vi "Bertta_v09_5.vi"() -> ()   [LabVIEW 2015]
uses:
  x64/Debug/BERTTA.dll
panel:
  out "TIME array":dbl[](array[numeric])
  out "TEMP array":dbl[](array[numeric])
  out "element":bool
  out "Started:":string
  in  "SHUTDOWN":bool
  in  "MASTER CONTROL":bool
  in  "Tab Control":T1(tab)
  in  "Read Seq":bool
  in  "Save Seq":bool
  in  "Configuration file":path=path "C:/Users/shresplab/Desktop/BerttaConfiguration.lvm" caption="Filename"
  in  "OK Button 2":bool
  out "Boolean":bool
  in  "User (initials)":string
  in  "Project name":string
  in  "Description":string
  out "Output file":string
  out "PUMP 3":bool
  out "Target amount":dbl
  out "Scale weight":dbl
  out "Amount now":dbl
  out "Flow rate":dbl
  out "Time to target":dbl format="%<%H:%M:%S>t"
  out "Current step":dbl
  out "Target amount":dbl
  out "Amount now":dbl
  out "Amount now":dbl
  out "Target amount":dbl
  out "Current step":dbl
  out "Time to target":dbl format="%<%H:%M:%S>t"
  out "Flow rate":dbl
  out "Amount now":dbl
  out "Scale weight":dbl
  out "Target amount":dbl
  out "PUMP 2":bool
  out "Sensor OK 6":bool
  out "Sensor OK 5":bool
  out "Sensor OK 4":bool
  out "Sensor OK 3":bool
  in  "OK Button":bool
  in  "Add comment":string
  out "PUMP 1":bool
  out "Target amount":dbl
  out "Scale weight":dbl
  out "Amount now":dbl
  out "Flow rate":dbl
  out "Time to target":dbl format="%<%H:%M:%S>t"
  out "Current step":dbl
  out "Target amount":dbl
  out "Amount now":dbl
  out "Tr":dbl
  out "Tj in":dbl
  out "Tj out":dbl
  out "T set":dbl
  out "Current step":i32
  out "RPM":dbl
  out "Torque 2":dbl
  out "Waveform Chart 5":dynamicdata(graph)
  out "Waveform Chart 6":dynamicdata(graph)
  out "Waveform Chart 7":dynamicdata(graph)
  in  "Tab Control 2":T2(tab)
  out "Waveform Chart 3":dynamicdata(graph)
  out "Waveform Chart 8":dynamicdata(graph)
  out "Waveform Chart 11":dynamicdata(graph)
  out "Waveform Chart 13":dynamicdata(graph)
  out "Waveform Chart 9":dynamicdata(graph)
  out "Table":string[][](table)=[["14.8.2017 18.06.59", "0,000000", "417,670000", "-0,150000", "1,000000", "22,220000", "23,366837", "23,574959", "23,985852", "23,690000", "240,000000", "4,000000", "0,000000", "397,000000", "-397,000000", "1,000000"], ["14.8.2017 18.07.06", "0,000000", "417,640000", "-0,120000", "1,000000", "22,220000", "23,763115", "23,906257", "23,985694", "23,680000", "240,000000", "4,000000", "0,000000", "397,000000", "-397,000000", "1,000000"], ["14.8.2017 18.07.13", "0,000000", "417,640000", "-0,120000", "1,000000", "22,220000", "23,965922", "24,013440", "23,984906", "23,670000", "240,000000", "4,100000", "3,000000", "397,000000", "-397,000000", "1,000000"], ["14.8.2017 18.07.21", "0,000000", "417,640000", "-0,120000", "1,000000", "22,220000", "23,943860", "23,900110", "23,987113", "23,670000", "240,000000", "4,000000", "0,000000", "397,000000", "-397,000000", "1,000000"], ["14.8.2017 18.07.28", "0,000000", "417,640000", "-0,120000", "1,000000", "22,220000", "23,736328", "23,600018", "23,989004", "23,660000", "240,000000", "4,000000", "0,000000", "397,000000", "-397,000000", "1,000000"], ["14.8.2017 18.07.36", "0,000000", "417,640000", "-0,120000", "1,000000", "22,220000", "23,480910", "23,324538", "23,991053", "23,660000", "240,000000", "4,000000", "0,000000", "397,000000", "-397,000000", "1,000000"], ["14.8.2017 18.07.43", "0,000000", "417,640000", "-0,120000", "2,000000", "22,220000", "23,195579", "23,008270", "23,999093", "23,650000", "240,000000", "4,000000", "0,000000", "397,000000", "-397,000000", "1,000000"], ["14.8.2017 18.07.51", "0,000000", "417,650000", "-417,650000", "1,000000", "22,220000", "22,862541", "22,649021", "24,003979", "23,650000", "240,000000", "4,000000", "0,000000", "397,000000", "-397,000000", "2,000000"], ["14.8.2017 18.07.58", "0,000000", "417,640000", "0,010000", "1,000000", "22,220000", "22,541353", "22,354878", "24,005398", "23,650000", "240,000000", "4,000000", "0,000000", "397,000000", "-397,000000", "1,000000"], ["14.8.2017 18.08.06", "0,000000", "417,640000", "0,010000", "1,000000", "22,220000", "22,347931", "22,253738", "24,007605", "23,640000", "240,000000", "4,100000", "0,000000", "397,000000", "-397,000000", "1,000000"], ["14.8.2017 18.08.13", "0,000000", "417,640000", "0,010000", "1,000000", "22,220000", "22,329030", "22,302102", "24,006028", "23,640000", "240,000000", "4,000000", "0,000000", "395,820000", "-395,820000", "1,000000"], ["14.8.2017 18.08.20", "0,000000", "417,640000", "0,010000", "1,000000", "22,220000", "22,466849", "22,511320", "24,002403", "23,630000", "240,000000", "4,000000", "0,000000", "395,830000", "-0,010000", "1,000000"], ["14.8.2017 18.08.28", "0,000000", "417,640000", "0,010000", "1,000000", "22,220000", "22,707062", "22,835101", "24,000984", "23,620000", "240,000000", "4,000000", "0,000000", "395,830000", "-0,010000", "1,000000"], ["14.8.2017 18.08.35", "0,000000", "417,640000", "0,010000", "1,000000", "22,220000", "23,054104", "23,232979", "24,001299", "23,600000", "240,000000", "4,000000", "0,000000", "395,830000", "-0,010000", "1,000000"], ["14.8.2017 18.08.43", "0,000000", "417,640000", "0,010000", "1,000000", "22,220000", "23,412371", "23,522793", "24,002560", "23,590000", "240,000000", "4,000000", "0,000000", "395,820000", "0,000000", "1,000000"], ["14.8.2017 18.08.51", "0,000000", "417,640000", "0,010000", "1,000000", "22,220000", "23,596247", "23,656125", "24,003821", "23,580000", "240,000000", "4,000000", "0,000000", "395,820000", "0,000000", "1,000000"]]
  in  "Reset":bool
  in  "Numeric 4":dbl=20.0
  in  "Numeric 3":dbl=30.0
  in  "Numeric 2":dbl=40.0
  in  "Numeric 1":dbl=30.0
  in  "Numeric":dbl=20.0
  out "Boolean 12":bool
  out "Boolean 7":bool
  out "Boolean 6":bool
  out "Boolean 5":bool
  out "Boolean 4":bool
  out "Boolean 19":bool
  in  "Numeric 5":dbl=5.0
  in  "Numeric 6":dbl=5.0
  in  "Numeric 7":dbl=5.0
  in  "Numeric 8":dbl=5.0
  in  "T ext / T ext 2":enum32{"External 1", "External 2"}(radio)
  out "Sensor OK":bool
  in  "T fail":dbl=20.0
  in  "?":bool
  in  "T manual setpoint":dbl=20.0
  in  "Lauda port":dbl=9.0
  in  "Manual select":enum32{"Tr", "Tj"}(radio)
  in  "PAUSE":bool
  out "Waveform Chart":dynamicdata(graph)
  out "T external 2":dbl
  out "result":bool
  in  "Port":i32=10
  in  "Radio Buttons 3":enum32{"Reglo Digital", "Reglo Analog", "PAM"}(radio)=enum."Reglo Analog"
  out "Speed":dbl
  out "mA":dbl format="%#_2g"
  in  "Port":i32=15
  out "RPM":dbl format="%#_2g"
  out "Led10 3":bool
  out "Led9 3":bool
  out "Led8 3":bool
  out "Led7 3":bool
  out "Led6 3":bool
  out "Led5 3":bool
  out "Led4 3":bool
  out "Led3 3":bool
  out "Led2 3":bool
  out "Led1 3":bool
  in  "PumpSeq 3":dbl[][](array[numeric])=[[0.0, 0.0, 7.0], [0.0, 0.0, 2.0], [0.0, 0.0, 100.0], [0.0, 0.0, 0.0], [0.0, 0.0, 0.0], [0.0, 0.0, 0.0], [0.0, 0.0, 0.0], [0.0, 0.0, 0.0], [0.0, 0.0, 0.0], [0.0, 0.0, 0.0], [0.0, 1.0, 0.0]]
  in  "?":bool
  out "Flow rate (g/min)":dbl
  out "Scale reading":dbl
  out "Step amount now":dbl
  out "Time to target":dbl format="%<%H:%M:%S>t"
  in  "Grams / min":dbl
  out "Waveform Chart 12":dynamicdata(graph)
  in  "?":bool
  out "Total amount now":dbl
  out "Total time 3":dbl
  out "Total amount target 3":dbl
  out "Led11 3":bool
  in  "Reset 4":bool
  in  "Port":i32=11
  in  "Radio Buttons 2":enum32{"Reglo Digital", "Reglo Analog", "PAM"}(radio)
  out "Speed":dbl
  out "mA":dbl format="%#_2g"
  in  "Port":i32=15
  out "RPM":dbl format="%_4f"
  out "Led10 2":bool
  out "Led9 2":bool
  out "Led8 2":bool
  out "Led7 2":bool
  out "Led6 2":bool
  out "Led5 2":bool
  out "Led4 2":bool
  out "Led3 2":bool
  out "Led2 2":bool
  out "Led1 2":bool
  in  "PumpSeq 2":dbl[][](array[numeric])=[[1.0, 2.0, 7.0], [2.0, 2.0, 2.0], [3.0, 2.0, 100.0], [0.0, 0.0, 0.0], [0.0, 0.0, 0.0], [0.0, 0.0, 0.0], [0.0, 0.0, 0.0], [0.0, 0.0, 0.0], [0.0, 0.0, 0.0], [0.0, 0.0, 0.0], [0.0, 1.0, 0.0]]
  in  "?":bool
  out "Flow rate (g/min)":dbl
  out "Scale reading":dbl
  out "Step amount now":dbl
  out "Time to target":dbl format="%<%H:%M:%S>t"
  in  "Grams / min":dbl
  out "Waveform Chart 10":dynamicdata(graph)
  in  "?":bool
  out "Total amount now":dbl
  out "Total time 2":dbl
  out "Total amount target 2":dbl
  out "Led11 2":bool
  in  "Reset 3":bool
  out "elapsed / step":i32
  out "step_fr":dbl
  in  "Port":i32=12
  in  "Radio Buttons":enum32{"Reglo Digital", "Reglo Analog", "PAM"}(radio)
  out "Speed":dbl
  out "mA":dbl format="%#_2g"
  in  "Port":i32=14
  out "RPM":dbl format="%#_2g"
  out "Led10":bool
  out "Led9":bool
  out "Led8":bool
  out "Led7":bool
  out "Led6":bool
  out "Led5":bool
  out "Led4":bool
  out "Led3":bool
  out "Led2":bool
  out "Led1":bool
  in  "PumpSeq":dbl[][](array[numeric])=[[0.0, 0.0, 7.0], [0.0, 0.0, 2.0], [0.0, 0.0, 100.0], [0.0, 0.0, 0.0], [0.0, 0.0, 0.0], [0.0, 0.0, 0.0], [0.0, 0.0, 0.0], [0.0, 0.0, 0.0], [0.0, 0.0, 0.0], [0.0, 0.0, 0.0], [0.0, 1.0, 0.0]]
  in  "?":bool
  out "Flow rate (g/min)":dbl
  out "Scale reading":dbl
  out "Step amount now":dbl
  out "Time to target":dbl format="%<%H:%M:%S>t"
  in  "Grams / min":dbl
  out "Waveform Chart 2":dynamicdata(graph)
  in  "?":bool
  out "Total amount now":dbl
  out "Total time":dbl
  out "Total amount target":dbl
  out "Led11":bool
  in  "Reset 2":bool
  in  "Bypass select 2":enum32{"Remote", "Manual"}(radio)=enum."Manual"
  in  "Port":dbl=13.0
  out "RPM":dbl
  out "Torque":dbl
  in  "Set RPM":dbl(slide) scale=0.0..2000.0
  out "Waveform Chart 4":dynamicdata(graph)
  in  "Cal pump 3":dbl=1.11
  in  "Cal pump 2":dbl=1.218 format="%#_13g"
  in  "Cal pump 1":dbl=1.0 format="%#_13g"
  out "DAQ 9217 (PT100)":errorcluster
  # "Temperature sensor:"
  # "Manual control:"
  # "PUMP & SCALE 1"
  # "STEP"
  # "TOTAL"
  # "PUMP & SCALE 2"
  # "STEP"
  # "TOTAL"
  # "PUMP & SCALE 3"
  # "STEP"
  # "TOTAL"
  # "Manual control"
  # "Secondary temperature sensor"
  # "Device communication"
  # "Temp"
  # "Time"
  # "Grams    /   min"
  # "End of sequence"
  # "Manual control"
  # "Device communication"
  # "Pump configuration"
  # "Scale configuration"
  # "SCALE 1"
  # "Grams    /   min"
  # "End of sequence"
  # "Manual control"
  # "Device communication"
  # "Pump configuration"
  # "Scale configuration"
  # "SCALE 2"
  # "Grams    /   min"
  # "End of sequence"
  # "Manual control"
  # "Device communication"
  # "Pump configuration"
  # "Scale configuration"
  # "SCALE 3"
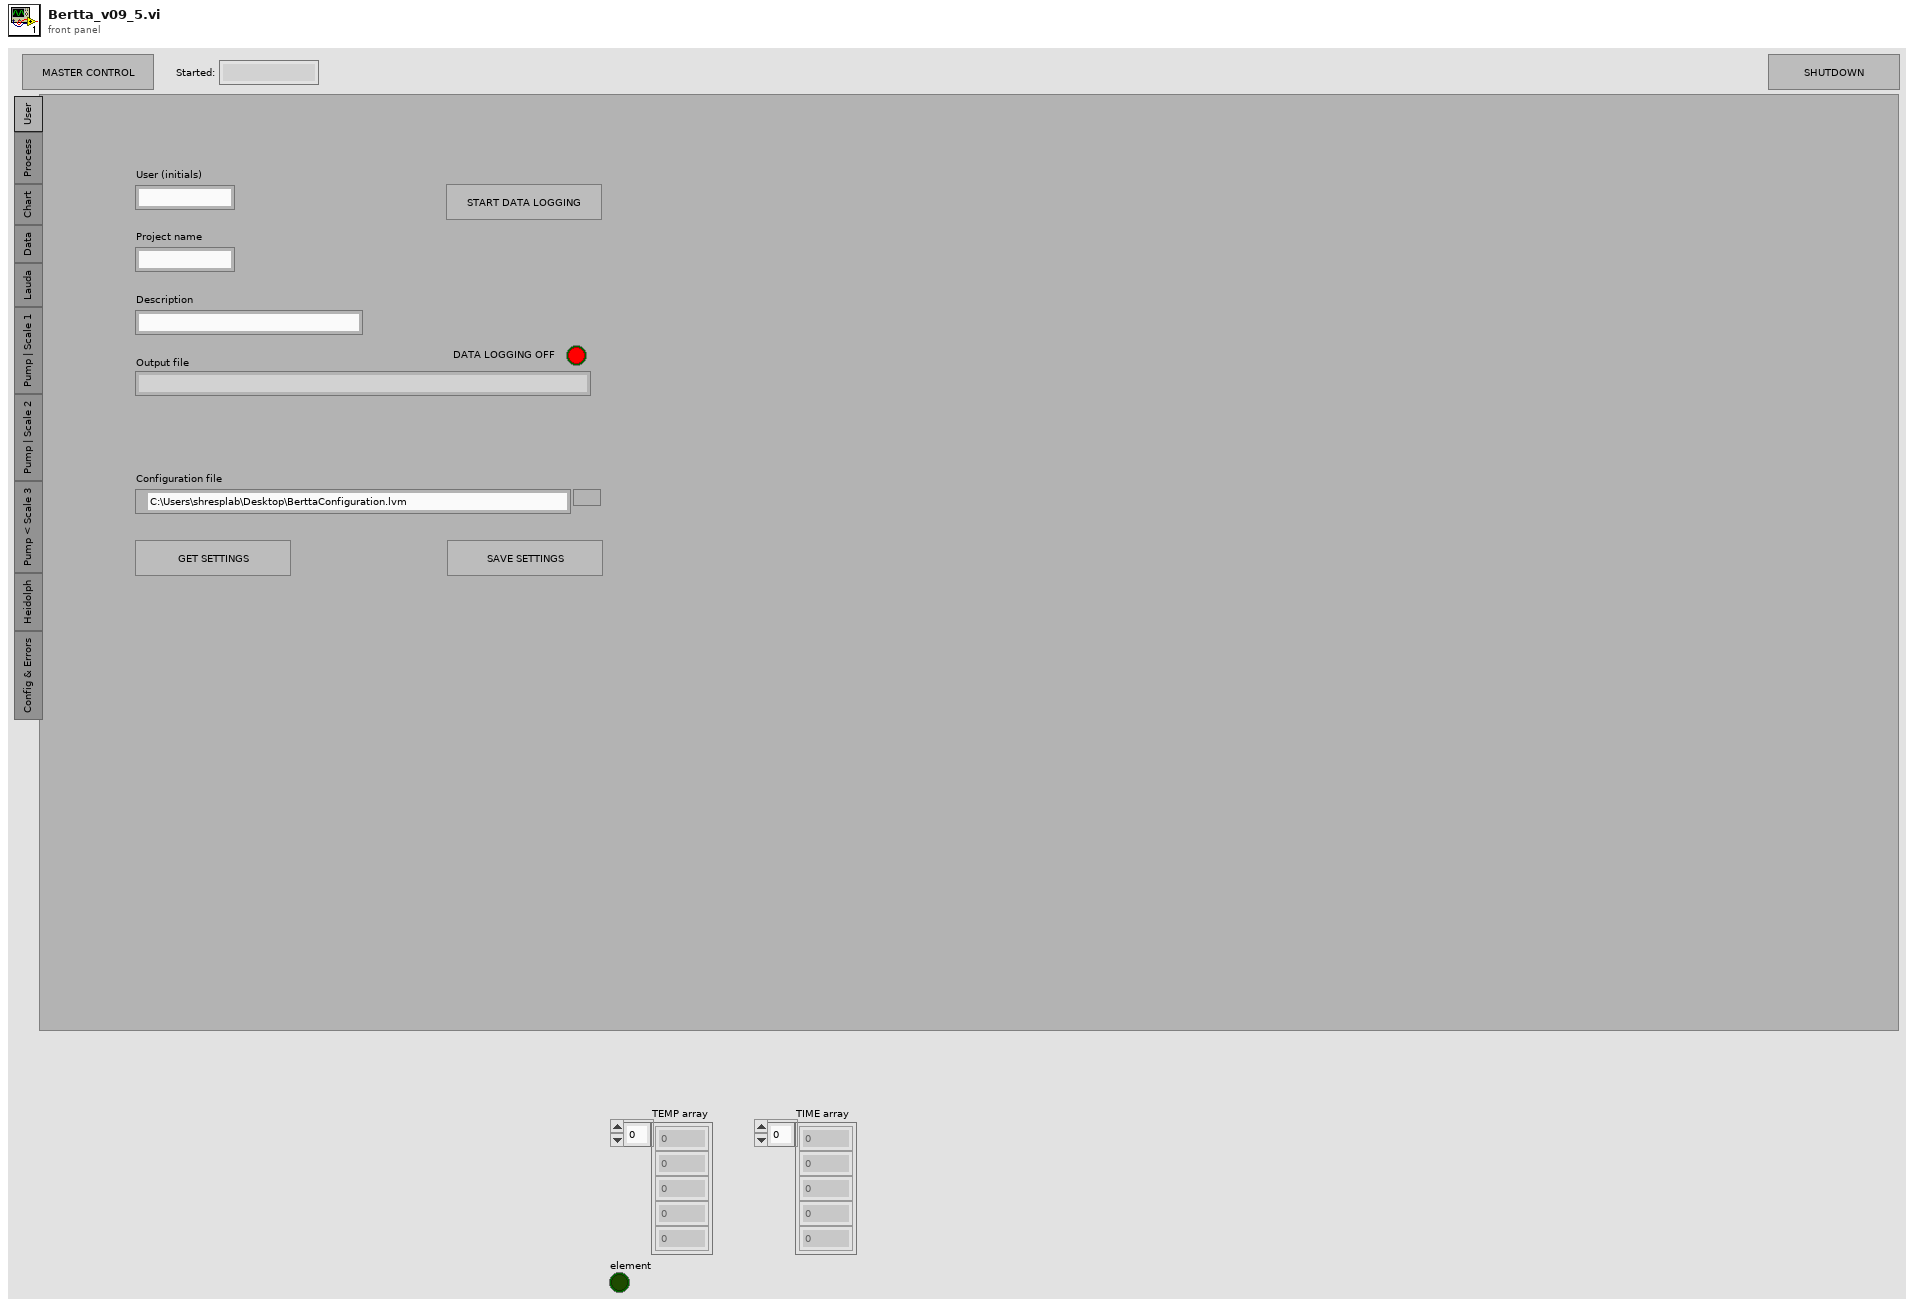
[diagram p1: front panel]
types:
  T1 = enum32{"User", "Process", "Chart", "Data", "Lauda", "Pump | Scale 1", "Pump | Scale 2", "Pump < Scale 3", "Heidolph", "Config & Errors"}
  T2 = enum32{"Temperatures", "Scale / Pump 1", "Scale / Pump 2", "Scale / Pump 3", "RPM / torque"}
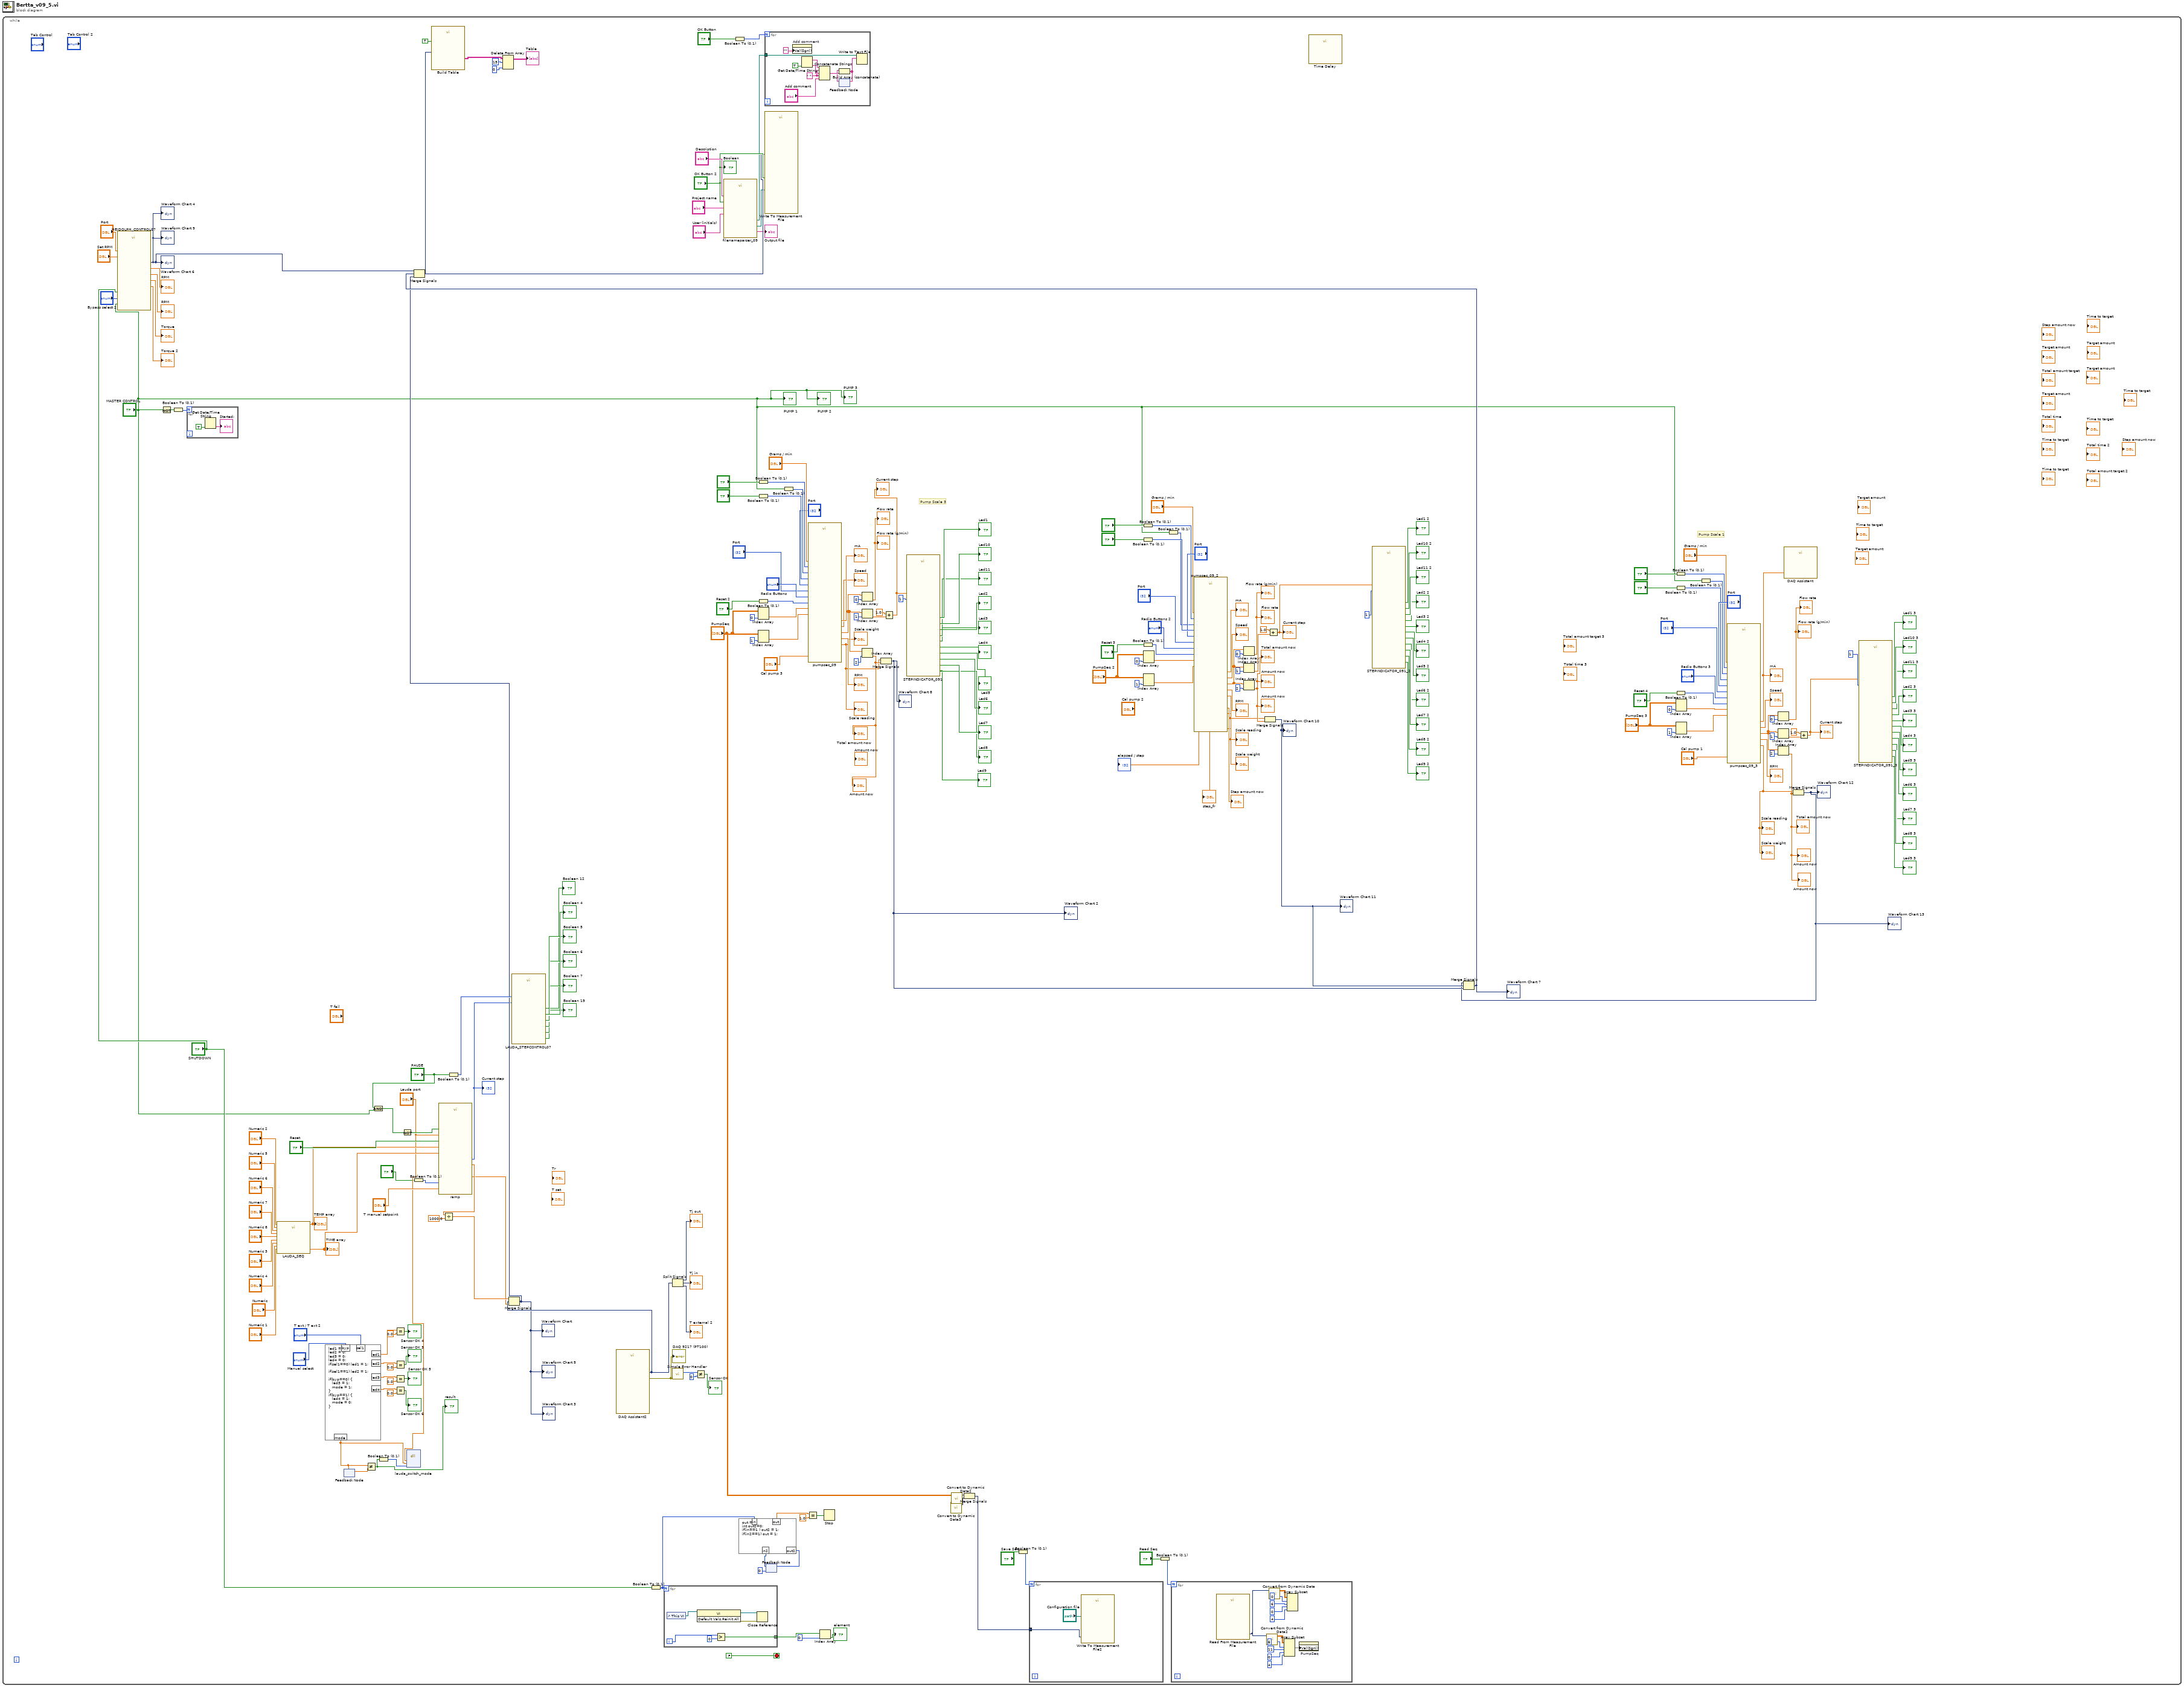
[diagram p0: block diagram]
diagram:
  n1 = while {
    stop <- FALSE stop-if-true
    # "Pump Scale 3"
    # "Pump Scale 1"
    n2 = call "HEIDOLPH_CONTROL07.vi"("master"="MASTER CONTROL", "shutdown"="SHUTDOWN", "Bypass select"="Bypass select 2", "Set RPM"="Set RPM", "Device port"="Port") -> ("Dynamic Data"=w229:dynamicdata, "RPM"=→"RPM":dbl, "RPM 2"=→"RPM":dbl, "Torque"=→"Torque":dbl, "Torque 2"=→"Torque 2":dbl)  [unwired: 2 in]
    "Waveform Chart 4" <- w229
    "Waveform Chart 6" <- w229
    "Waveform Chart 9" <- w229
    n3 = Not(x="MASTER CONTROL") -> (.not. x?=w214:bool)
    n4 = Boolean To (0,1)(Boolean=w214) -> (0, 1=w215:i16)
    n5 = for {
      N: w215 -> [_]
      n6 = Get Date/Time String(want seconds? (F)=TRUE) -> (time string=→"Started:":string)  [unwired: 2 in, 1 out]
    }
    n7 = call "LAUDA_SEQ.vi"("Numeric 2"="Numeric 2", "Numeric 1"="Numeric 1", "Numeric"="Numeric", "Numeric 5"="Numeric 5", "Numeric 6"="Numeric 6", "Numeric 7"="Numeric 7", "Numeric 8"="Numeric 8", "Numeric 3"="Numeric 3", "Numeric 4"="Numeric 4") -> ("output array"=w16:dbl[], "output array 2"=w15:dbl[])  [unwired: 5 in]
    "TEMP array" <- w16
    "TIME array" <- w15
    n8 = formula code="led1 = 0;\nled2 = 0;\nled3 = 0;\nled4 = 0;\nif(sel1==0) led1 = 1;\n\nif(sel1==1) led2 = 1;\n\nif(byp==0) {\n   led3 = 1;\n   mode = 1;\n}\nif(byp==1) {\n   led4 = 1;\n   mode = 0;\n}"("sel1"="T ext / T ext 2", "byp"="Manual select") -> ("led1"=w184:dbl, "led2"=w182:dbl, "led3"=w177:dbl, "led4"=w176:dbl, "mode"=w9:dbl)
    n9 = feedback-in #1(w9) -> ()
    n10 = feedback #1() -> (w8:dbl)  [unwired: 1 in]
    n11 = Not Equal?(x=w9, y=w8) -> (x != y?=w6:bool)
    "result" <- w6
    n12 = And(x="PAUSE", y="MASTER CONTROL") -> (x .and. y?=w28:bool)
    n13 = Boolean To (0,1)(Boolean=w6) -> (0, 1=w7:i16)
    n14 = Equal?(x=w184, y=0.0) -> (x = y?=→"Sensor OK 4":bool)
    n15 = Equal?(x=w182, y=0.0) -> (x = y?=→"Sensor OK 3":bool)
    n16 = Equal?(x=w177, y=0.0) -> (x = y?=→"Sensor OK 5":bool)
    n17 = Equal?(x=w176, y=0.0) -> (x = y?=→"Sensor OK 6":bool)
    n18 = Not(x=w28) -> (.not. x?=w27:bool)
    n19 = dll-call lib="C:/Users/shresplab/OneDrive - Kemira Oyj/Documents/Visual Studio 2017/Projects/Bertta/BERTTA/x64/Debug/BERTTA.dll" fn="lauda_switch_mode"("port"="Lauda port", "mode"=w9, "enable"=w7) -> ()  [unwired: 7 in, 2 out]
    n20 = Boolean To (0,1)(Boolean="?") -> (0, 1=w12:i16)
    n21 = call "ramp.vi"("TimeParams"=w15, "Seq"=w16, "T_man"="T manual setpoint", "manual"=w12, "port"="Lauda port", "reset"="Reset", "pause"=w27) -> ("T control"=w32:dbl, "STEP"=w34:i32, "T ext"=w14:dbl)  [unwired: 1 in, 1 out]
    "Current step" <- w34
    n22 = Divide(x=w32, y=1000.0) -> (x/y=w31:dbl)
    n23 = Boolean To (0,1)(Boolean="PAUSE") -> (0, 1=w171:i16)
    n24 = call "LAUDA_STEPCONTROL07.vi"("step"=w34, "pause"=w171) -> ("Boolean 13"=→"Boolean 19":bool, "Boolean 6"=→"Boolean 6":bool, "Boolean 5"=→"Boolean 5":bool, "Boolean 4"=→"Boolean 4":bool, "Boolean 7"=→"Boolean 7":bool, "Boolean 12"=→"Boolean 12":bool)  [unwired: 4 in]
    n25 = call "DAQ Assistant2"() -> ("data"=w54:dynamicdata, "error out"=w224:errorcluster)  [unwired: 17 in, 1 out]
    "DAQ 9217 (PT100)" <- w224
    n26 = Merge Signals(w31, w54, w14) -> (w51:dynamicdata)
    "Waveform Chart 3" <- w51
    "Waveform Chart" <- w51
    "Waveform Chart 5" <- w51
    n27 = Boolean To (0,1)(Boolean="SHUTDOWN") -> (0, 1=w189:i16)
    n28 = for {
      N: w189 -> [_]
      tunnel: [w260] -> w213 mode=indexing
      i -> [w262]
      n29 = control-ref of="This VI"() -> (w265:refnum<vi>)
      n30 = invoke class="VI" method="Default Vals.Reinit All"(reference=w265) -> (reference out=w263:refnum<vi>, error out=w264:errorcluster)  [unwired: 2 in, 1 out]
      n31 = Greater?(x=w262, y=0) -> (0:w260:bool)
      n32 = Close Reference(reference=w263, error in (no error)=w264) -> ()  [unwired: 1 out]
    }
    n33 = Split Signals(w54) -> (→"Tj out":dynamicdata, →"Tj in":dynamicdata, →"T external 2":dynamicdata)  [unwired: 3 in]
    n34 = call <vilib>:"Simple Error Handler.vi"("error in (no error)"=w224) -> ("code out"=w223:i32)  [unwired: 4 in, 4 out]
    n35 = Not Equal?(x=w223, y=0) -> (x != y?=→"Sensor OK":bool)
    n36 = call "filenameparser_09.vi"("Description"="Description", "Project name"="Project name", "User (initials)"="User (initials)", "OK Button in"="OK Button 2") -> ("Output file"=→"Output file":string, "appended path 2"=w196:path, "appended path"=w195:path)  [unwired: 5 in]
    n37 = Boolean To (0,1)(Boolean="OK Button") -> (0, 1=w194:i16)
    n38 = Boolean To (0,1)(Boolean="?") -> (0, 1=w160:i16)
    n39 = Boolean To (0,1)(Boolean="?") -> (0, 1=w156:i16)
    n40 = Boolean To (0,1)(Boolean="Reset 2") -> (0, 1=w158:i16)
    n41 = Index Array(array="PumpSeq", index (col)=0 ("disabled index (col)")) -> (element=w165:dbl[])  [unwired: 1 in]
    n42 = Index Array(array="PumpSeq", index (col)=1 ("disabled index (col)")) -> (element=w164:dbl[])  [unwired: 1 in]
    n43 = for {
      N: w194 -> [_]
      tunnel: w195 -> [w238]
      w242 = " " ("string")
      n44 = property on="Add comment" class="Str"("Val(Sgnl)"="" ("Value (Signaling)")) -> ()  [unwired: 2 in, 2 out]
      n45 = Get Date/Time String(want seconds? (F)=TRUE) -> (date string=w245:string, time string=w243:string)  [unwired: 2 in]
      n46 = Concatenate Strings(w245, w242, w243, w242, "Add comment") -> (w241:string)
      n47 = feedback #2() -> (w240:string[])  [unwired: 1 in]
      n48 = Build Array (concatenate)(w240, w241) -> (w239:string[])
      n49 = feedback-in #2(w239) -> ()
      n50 = Write to Text File(file (use dialog)=w238, text=w239) -> ()  [unwired: 2 in, 3 out]
    }
    n51 = feedback #3(0) -> (w187:i32)
    n52 = formula code="out = 0;\nint out2=0;\nif(in==1 ) out2 = 1;\nif(in2==1) out = 1;"("in"=w189, "in2"=w187) -> ("out"=w191:dbl, "out2"=w188:i32)
    n53 = feedback-in #3(w188) -> ()
    n54 = Boolean To (0,1)(Boolean="MASTER CONTROL") -> (0, 1=w155:i16)
    n55 = Equal?(x=w191, y=1.0) -> (x = y?=w190:bool)
    n56 = call "pumpsec_09.vi"("reset"=w158, "master"=w155, "correction"="Cal pump 3", "manual"=w160, "pause"=w156, "Port"="Port", "pump_type"="Radio Buttons", "port, Reglo D"="Port", "Target"=w165, "Time"=w164, "fr_manual"="Grams / min") -> ("Reglo D"=→"RPM":dbl, "Scale"=w93:dbl, "mA"=→"mA":dbl, "params"=w147:dbl[], "PAM"=→"Speed":dbl)  [unwired: 3 in, 1 out]
    "Scale reading" <- w93
    "Scale weight" <- w93
    n57 = Index Array(array=w213, index=0) -> (element=→"element":bool)
    n58 = Stop(stop? (T)=w190) -> ()
    n59 = Index Array(array=w147, index=0) -> (element=→"Flow rate (g/min)" →"Flow rate":dbl)
    n60 = Index Array(array=w147, index=1) -> (element=w149:dbl)
    n61 = Index Array(array=w147, index=2) -> (element=w129:dbl)
    "Total amount now" <- w129
    "Amount now" <- w129
    n62 = Merge Signals(w93, w129) -> (w53:dynamicdata)
    "Waveform Chart 2" <- w53
    "Waveform Chart 8" <- w53
    n63 = Add(x=1.0, y=w149) -> (x+y=w131:dbl)
    "Current step" <- w131
    n64 = call "STEPINDICATOR_091.vi"("current step"=w131, "enable"=i16 1) -> ("Led 8"=→"Led8":bool, "Led 10"=→"Led10":bool, "Led 11"=→"Led11":bool, "Led 7"=→"Led7":bool, "Led 1"=→"Led1":bool, "Led 6"=→"Led6":bool, "Led 2"=→"Led2":bool, "Led 5"=→"Led5":bool, "Led 4"=→"Led4":bool, "Led 3"=→"Led3":bool, "Led 9"=→"Led9":bool)  [unwired: 3 in]
    n65 = call "Convert to Dynamic Data3"() -> ("Dynamic Data Type"=w173:dynamicdata)  [unwired: 4 in]
    n66 = call "Convert to Dynamic Data2"("2D Array"="PumpSeq") -> ("Dynamic Data Type"=w211:dynamicdata)  [unwired: 3 in]
    n67 = Merge Signals(w211, w173) -> (w210:dynamicdata)
    n68 = Boolean To (0,1)(Boolean="Save Seq") -> (0, 1=w209:i16)
    n69 = for {
      N: w209 -> [_]
      tunnel: w210 -> [w259]
      n70 = call "Write To Measurement File2"("Signals"=w259, "Filename"="Configuration file") -> ()  [unwired: 15 in, 3 out]
    }
    n71 = Boolean To (0,1)(Boolean="?") -> (0, 1=w37:i16)
    n72 = Boolean To (0,1)(Boolean="?") -> (0, 1=w122:i16)
    n73 = Boolean To (0,1)(Boolean="Reset 3") -> (0, 1=w119:i16)
    n74 = Index Array(array="PumpSeq 2", index (col)=0 ("disabled index (col)")) -> (element=w125:dbl[])  [unwired: 1 in]
    n75 = Index Array(array="PumpSeq 2", index (col)=1 ("disabled index (col)")) -> (element=w124:dbl[])  [unwired: 1 in]
    n76 = Boolean To (0,1)(Boolean="Read Seq") -> (0, 1=w206:i16)
    n77 = Boolean To (0,1)(Boolean="MASTER CONTROL") -> (0, 1=w112:i16)
    n78 = for {
      N: w206 -> [_]
      n79 = call "Read From Measurement File"() -> ("Signals"=w248:dynamicdata)  [unwired: 6 in, 5 out]
      n80 = call "Convert from Dynamic Data2"("Dynamic Data Type"=w248) -> ("Array"=w247:dbl[][])  [unwired: 3 in]
      n81 = call "Convert from Dynamic Data"("Dynamic Data Type"=w248) -> ("Array"=w255:dbl[][])  [unwired: 3 in]
      n82 = Array Subset(array=w247, index (row)=6 ("index"), length (row)=11 ("length"), index (col)=0 ("index"), length (col)=4 ("length")) -> (w246:dbl[][])
      n83 = Array Subset(array=w255, index (row)=0 ("index"), length (row)=6 ("length"), index (col)=0 ("index"), length (col)=4 ("length")) -> ()  [unwired: 1 out]
      n84 = property on="PumpSeq" class="Arr (strict)"("Val(Sgnl)"=w246) -> ()  [unwired: 2 in, 2 out]
    }
    n85 = call "pumpsec_09_2.vi"("reset"=w119, "master"=w112, "manual"=w37, "pause"=w122, "Port"="Port", "pump_type"="Radio Buttons 2", "port, Reglo D"="Port", "Target"=w125, "fr_manual"="Grams / min", "Time"=w124) -> ("step_fr"=→"step_fr":dbl, "amount_step"=→"Step amount now":dbl, "Reglo D"=→"RPM":dbl, "Scale"=w4:dbl, "mA"=→"mA":dbl, "elapsed_step"=→"elapsed / step":dbl, "params"=w113:dbl[], "PAM"=→"Speed":dbl)  [unwired: 8 in, 2 out]
    "Scale weight" <- w4
    "Scale reading" <- w4
    n86 = Index Array(array=w113, index=0) -> (element=→"Flow rate" →"Flow rate (g/min)":dbl)
    n87 = Index Array(array=w113, index=1) -> (element=w116:dbl)
    n88 = Index Array(array=w113, index=2) -> (element=w39:dbl)
    "Amount now" <- w39
    "Amount now" <- w39
    "Total amount now" <- w39
    n89 = Merge Signals(w4, w39) -> (w52:dynamicdata)
    "Waveform Chart 11" <- w52
    "Waveform Chart 10" <- w52
    n90 = Add(x=1.0, y=w116) -> (x+y=w105:dbl)
    "Current step" <- w105
    n91 = call "Time Delay"() -> ()  [unwired: 11 in, 1 out]
    n92 = call "STEPINDICATOR_091_2.vi"("current step"=w105, "enable"=i16 1) -> ("Led 8"=→"Led8 2":bool, "Led 10"=→"Led10 2":bool, "Led 11"=→"Led11 2":bool, "Led 7"=→"Led7 2":bool, "Led 1"=→"Led1 2":bool, "Led 6"=→"Led6 2":bool, "Led 2"=→"Led2 2":bool, "Led 5"=→"Led5 2":bool, "Led 4"=→"Led4 2":bool, "Led 3"=→"Led3 2":bool, "Led 9"=→"Led9 2":bool)  [unwired: 3 in]
    n93 = Boolean To (0,1)(Boolean="?") -> (0, 1=w86:i16)
    n94 = Boolean To (0,1)(Boolean="?") -> (0, 1=w72:i16)
    n95 = Boolean To (0,1)(Boolean="Reset 4") -> (0, 1=w58:i16)
    n96 = Index Array(array="PumpSeq 3", index (col)=0 ("disabled index (col)")) -> (element=w81:dbl[])  [unwired: 1 in]
    n97 = Index Array(array="PumpSeq 3", index (col)=1 ("disabled index (col)")) -> (element=w80:dbl[])  [unwired: 1 in]
    n98 = Boolean To (0,1)(Boolean="MASTER CONTROL") -> (0, 1=w85:i16)
    n99 = call "pumpsec_09_3.vi"("reset"=w58, "master"=w85, "correction"="Cal pump 1", "manual"=w86, "pause"=w72, "Port"="Port", "pump_type"="Radio Buttons 3", "port, Reglo D"="Port", "Target"=w81, "fr_manual"="Grams / min", "Time"=w80) -> ("Reglo D"=→"RPM":dbl, "Scale"=w47:dbl, "mA"=w57:dbl, "params"=w77:dbl[], "PAM"=→"Speed":dbl)  [unwired: 3 in, 1 out]
    "Scale reading" <- w47
    "mA" <- w57
    "Scale weight" <- w47
    n100 = Index Array(array=w77, index=0) -> (element=→"Flow rate (g/min)" →"Flow rate":dbl)
    n101 = Index Array(array=w77, index=1) -> (element=w79:dbl)
    n102 = Index Array(array=w77, index=2) -> (element=w49:dbl)
    "Total amount now" <- w49
    "Amount now" <- w49
    "Amount now" <- w49
    n103 = call "DAQ Assistant"("data"=w57) -> ()  [unwired: 17 in, 2 out]
    n104 = Merge Signals(w47, w49) -> (w50:dynamicdata)
    "Waveform Chart 12" <- w50
    "Waveform Chart 13" <- w50
    n105 = Merge Signals(w50, w52, w53) -> (w55:dynamicdata)
    "Waveform Chart 7" <- w55
    n106 = Merge Signals(w229, w55, w51) -> (w201:dynamicdata)
    n107 = call "Build Table"("Include time data"=TRUE, "Signals"=w201) -> ("Table"=w200:string[][])  [unwired: 3 in, 6 out]
    n108 = Delete From Array(array=w200, length=15, index (col)=0 ("index (row)")) -> (array with subset deleted=→"Table":string[][])  [unwired: 1 in, 1 out]
    n109 = call "Write To Measurement File"("Signals"=w201, "Enable"="OK Button 2", "Filename"=w196) -> ()  [unwired: 14 in, 3 out]
    n110 = Add(x=1.0, y=w79) -> (x+y=w48:dbl)
    "Current step" <- w48
    n111 = call "STEPINDICATOR_091_3.vi"("current step"=w48, "enable"=i16 1) -> ("Led 8"=→"Led8 3":bool, "Led 10"=→"Led10 3":bool, "Led 11"=→"Led11 3":bool, "Led 7"=→"Led7 3":bool, "Led 1"=→"Led1 3":bool, "Led 6"=→"Led6 3":bool, "Led 2"=→"Led2 3":bool, "Led 5"=→"Led5 3":bool, "Led 4"=→"Led4 3":bool, "Led 3"=→"Led3 3":bool, "Led 9"=→"Led9 3":bool)  [unwired: 3 in]
    "PUMP 1" <- "MASTER CONTROL"
    "Boolean" <- "OK Button 2"
    "PUMP 2" <- "MASTER CONTROL"
    "PUMP 3" <- "MASTER CONTROL"
  }
